vi "BRig_dataTrial_Cue_n.vi"() -> (2 "output_Cue_n":i32)   [LabVIEW 2014]
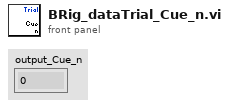
[diagram p1: front panel]
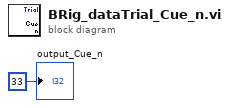
[diagram p0: block diagram]
diagram:
  "output_Cue_n" <- 33 ("output_iBlock")
